vi "Set Y Epsilon.vi"(8 "error in (no error)":errorcluster, 10 "Value":dbl, 11 "QR Code Detector in":refnum<class "QR Code Detector.lvclass">) -> (0 "error out":errorcluster, 3 "QR Code Detector":refnum<class "QR Code Detector.lvclass">)   [LabVIEW 2020, in "feature_detection.lvlib" / "QR Code Detector.lvclass"]
doc: "Adjust the Y Epsilon factor when decoding pixels of the QR Code."
uses:
  QR Code Detector.lvclass
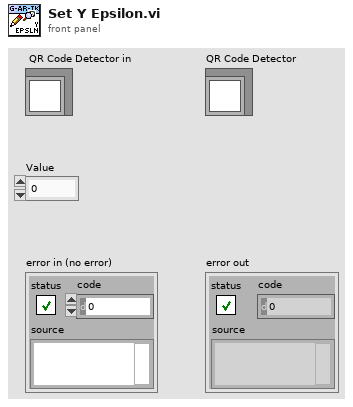
[diagram p1: front panel]
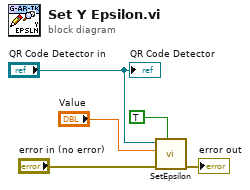
[diagram p0: block diagram]
diagram:
  n1 = call "SetEpsilon.vi"("y?"=TRUE, "error in (no error)"="error in (no error)", "Value in"="Value", "QR Code Detector in"="QR Code Detector in") -> ("error out"=→"error out":errorcluster)  [unwired: 7 in]
  "QR Code Detector" <- "QR Code Detector in"
